vi "Configure PRACH Modulation Result Enabled.vi"(4 "Modulation IQ (Off)":bool, 5 "Phase Error (Off)":bool, 6 "Magnitude Error (Off)":bool, 7 "EVM Vs Preamble (Off)":bool, 8 "error in (no error)":errorcluster, 9 "EVM (On)":bool=TRUE, 10 "Instance (1)":T1=1, 11 "VISA resource name":refnum<visa-resource-name>) -> (0 "error out":errorcluster, 3 "VISA resource name out":refnum<visa-resource-name>)   [LabVIEW 2020, in "Rohde&Schwarz CMWXP NR FR1 Measurement.lvlib"]
doc: "Enables or disables the evaluation of results in the PRACH measurement.\n\nAttributes:\nRSCMWXPNRFR1M_ATTR_PRACH_MODULATION_EVM_RESULT_ENABLED\nRSCMWXPNRFR1M_ATTR_PRACH_MODULATION_EVM_VS_PREAMBLE_RESULT_ENABLED\nRSCMWXPNRFR1M_ATTR_PRACH_MODULATION_MAGNITUDE_ERROR_RESULT_ENABLED\nRSCMWXPNRFR1M_ATTR_PRACH_MODULATION_PHASE_ERROR_RESULT_ENABLED\nRSCMWXPNRFR1M_ATTR_PRACH_MODULATION_IQ_RESULT_ENABLED\n\nRemote-control commands:\nCONFigure:NRSub:MEAS<i>:PRACh:RESult:EVMagnitude\nCONFigure:NRSub:MEAS<i>:PRACh:RESult:EVPReamble\nCONFigure:NRSub:MEAS<i>:PRACh:RESult:MERRor\nCONFigure:NRSub:MEAS<i>:PRACh:RESult:PERRor\nCONFigure:NRSub:MEAS<i>:PRACh:RESult:IQ"
uses:
  <instrlib>/Rohde&Schwarz CMWXP NR FR1 Measurement/Rohde&Schwarz CMWXP NR FR1 Measurement.lvlib
  <instrlib>/Rohde&Schwarz CMWXP NR FR1 Measurement/Private/_Instance.ctl
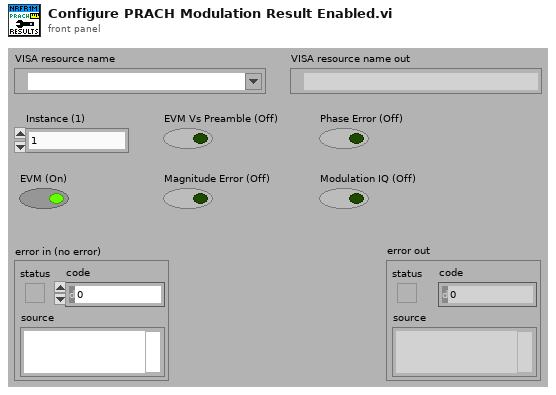
[diagram p1: front panel]
types:
  T1 = typedef "Rohde&Schwarz CMWXP NR FR1 Measurement.lvlib/_Instance.ctl" = i32
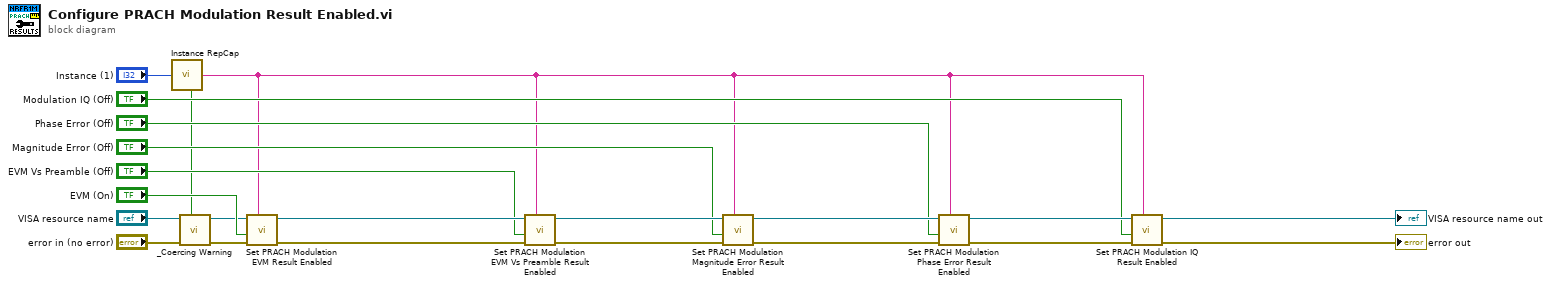
[diagram p0: block diagram]
diagram:
  n1 = call <instrlib>:"Instance RepCap.vi"("Instance In"="Instance (1)") -> ("In Range?"=w2:bool, "RepCap Identifier Out"=w1:string)  [unwired: 1 in]
  n2 = call <instrlib>:"_Coercing Warning.vi"("In Range?"=w2, "error in (no error)"="error in (no error)", "VISA resource name"="VISA resource name") -> ("error out"=w5:errorcluster, "VISA resource name out"=w4:refnum<visa-resource-name>)  [unwired: 7 in]
  n3 = call "Set PRACH Modulation EVM Result Enabled"("Repeated Capabilities"=w1, "error in (no error)"=w5, "PRACH Modulation EVM Result Enabled (OFF)"="EVM (On)", "instrument handle"=w4) -> ("error out"=w20:errorcluster, "instrument handle out"=w21:refnum<visa-resource-name>)  [unwired: 6 in]
  n4 = call "Set PRACH Modulation EVM Vs Preamble Result Enabled"("Repeated Capabilities"=w1, "error in (no error)"=w20, "PRACH Modulation EVM Vs Preamble Result Enabled (OFF)"="EVM Vs Preamble (Off)", "instrument handle"=w21) -> ("error out"=w17:errorcluster, "instrument handle out"=w18:refnum<visa-resource-name>)  [unwired: 6 in]
  n5 = call "Set PRACH Modulation Magnitude Error Result Enabled"("Repeated Capabilities"=w1, "error in (no error)"=w17, "PRACH Modulation Magnitude Error Result Enabled (OFF)"="Magnitude Error (Off)", "instrument handle"=w18) -> ("error out"=w14:errorcluster, "instrument handle out"=w15:refnum<visa-resource-name>)  [unwired: 6 in]
  n6 = call "Set PRACH Modulation Phase Error Result Enabled"("Repeated Capabilities"=w1, "error in (no error)"=w14, "PRACH Modulation Phase Error Result Enabled (OFF)"="Phase Error (Off)", "instrument handle"=w15) -> ("error out"=w9:errorcluster, "instrument handle out"=w10:refnum<visa-resource-name>)  [unwired: 6 in]
  n7 = call "Set PRACH Modulation IQ Result Enabled"("Repeated Capabilities"=w1, "error in (no error)"=w9, "PRACH Modulation IQ Result Enabled (OFF)"="Modulation IQ (Off)", "instrument handle"=w10) -> ("error out"=→"error out":errorcluster, "instrument handle out"=→"VISA resource name out":refnum<visa-resource-name>)  [unwired: 6 in]
